vi "Write Controller Enqueuer.vi"(10 "控制器待入队列":refnum<class "Message Enqueuer.lvclass">, 11 "冷却器输入":refnum<class "Cooler.lvclass">) -> (3 "冷却器输出":refnum<class "Cooler.lvclass">)   [LabVIEW 2015, in "Cooler.lvlib" / "Cooler.lvclass"]
doc: "写入向控制器发送消息的待入队列。如将输入设置为“非法引用句柄”待入队列，则表示冷却器当前不受任何控制器的控制。"
uses:
  Cooler.lvclass
  <vilib>/ActorFramework/Message Enqueuer/Message Enqueuer.lvclass
  Cooler.lvclass/Cooler.ctl
  <vilib>/ActorFramework/Message Enqueuer/Message Priority.ctl
  Cooler Controller/Update Current Temperature Msg/Update Current Temperature Msg.lvclass/Update Current Temperature Msg.ctl
  <vilib>/ActorFramework/Message Enqueuer/Message Enqueuer.lvclass/Message Enqueuer.ctl
  <vilib>/ActorFramework/Message Enqueuer/Enqueue.vi
  <vilib>/ActorFramework/Message Priority Queue/Priority Enqueue.vi
  Cooler Controller/Update Current Temperature Msg/Update Current Temperature Msg.lvclass
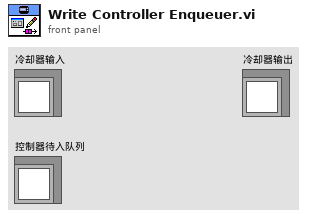
[diagram p1: front panel]
types:
  T1 = typedef "Actor Framework.lvlib/Message Enqueuer.lvclass/Message Priority.ctl" = enum16{"Low", "Normal", "High"}
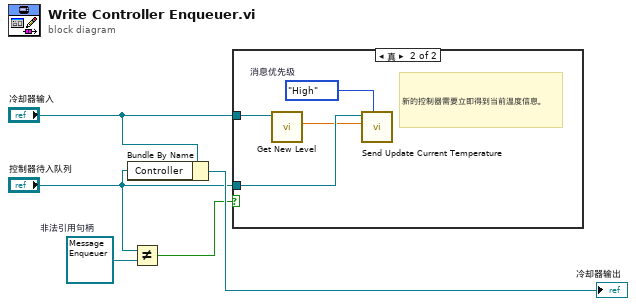
[diagram p0: block diagram]
diagram:
  w4 = refnum<class "Message Enqueuer.lvclass"> refnum  # 非法引用句柄
  n1 = Bundle By Name(cluster="冷却器输入", "Controller"="控制器待入队列") -> (→"冷却器输出":refnum<class "Cooler.lvclass">)
  n2 = Not Equal?(x="控制器待入队列", y=w4) -> (x != y?=w3:bool)
  n3 = case shown="真" w3 {
    tunnel: "控制器待入队列" -> [_ w9]
    tunnel: "冷却器输入" -> [_ w7]
    frame False {
    }
    frame True {
      w6 = Message_Priority."High"  # 消息优先级
      # "新的控制器需要立即得到当前温度信息。"
      n4 = call-dynamic "Get New Level.vi"("冷却器输入"=w7) -> ("水位"=w8:dbl)  [unwired: 8 in, 2 out]
      n5 = call "Send Update Current Temperature.vi"("消息优先级（标准）"=w6, "当前温度"=w8, "消息待入队列"=w9) -> ()  [unwired: 8 in, 1 out]
    }
  }
